vi "Trace Message.vi"(8 "error in (no error)":errorcluster, 10 "Message":string, 11 "XBoxController in":refnum<class "XBoxController.lvclass">) -> (0 "error out":errorcluster, 3 "XBoxController out":refnum<class "XBoxController.lvclass">)   [LabVIEW 2013, in "XBoxController.lvclass"]
uses:
  XBoxController.lvclass
  XBoxController.lvclass/XBoxController.ctl
  TraceMessage/Trace.lvclass
  System/System.lvclass
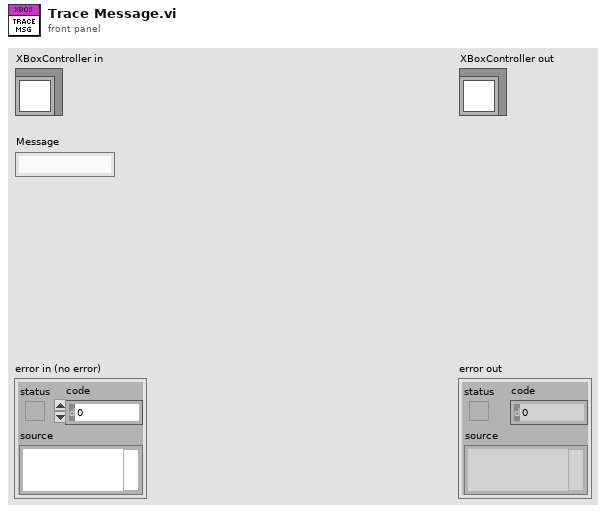
[diagram p1: front panel]
types:
  T1 = cluster{"Left Bumper":bool, "Right Bumper":bool, "Left Joystick Forward":dbl, "Left Joystick Right":dbl, "Right Joystick Forward":dbl, "Right Joystick Right":dbl}
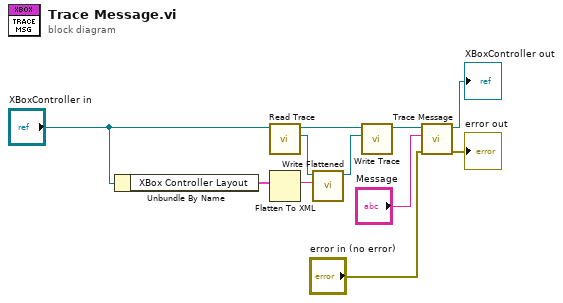
[diagram p0: block diagram]
diagram:
  n1 = Unbundle By Name("XBoxController in") -> ("XBox Controller Layout"=w3:T1)
  n2 = call-dynamic "Read Trace.vi"("System in"="XBoxController in") -> ("Trace.lvclass"=w1:refnum<class "Trace.lvclass">, "System out"=w7:refnum<class "XBoxController.lvclass">)  [unwired: 8 in, 1 out]
  n3 = Flatten To XML(anything=w3) -> (xml string=w2:string)
  n4 = call-dynamic "Write Flattened.vi"("Flattened"=w2, "TraceMessage in"=w1) -> ("TraceMessage out"=w6:refnum<class "Trace.lvclass">)  [unwired: 8 in, 1 out]
  n5 = call-dynamic "Write Trace.vi"("Trace.lvclass"=w6, "System in"=w7) -> ("System out"=w5:refnum<class "XBoxController.lvclass">)  [unwired: 8 in, 1 out]
  n6 = call-parent "Trace Message.vi"("error in (no error)"="error in (no error)", "Message"="Message", "System in"=w5) -> ("error out"=→"error out":errorcluster, "System out"=→"XBoxController out":refnum<class "XBoxController.lvclass">)  [unwired: 7 in]
